vi "SweepCtrlConstCurrent_ver1.0.vi"(7 "Keithley 6221":T1={"Delta "=FALSE, "Const I "=FALSE, "Pulse Delta "=FALSE, "Sine Wave "=FALSE, "From I_HI (A)"=0.0, "From I (A)"=0.0, "I_LO (A)"=0.0, "From I_H (A)"=0.0, "I_L (A)"=0.0, "Freq (Hz)"=13.259, "From I_Sin (A)"=0.0, "DC Offset (A)"=0.0, "Delay Time (s)"=1.0, "Pulse Width (s)"=0.012, "Delay (s)"=0.011966, "To I (A)"=0.0, "ASymmetric?"=FALSE, "To I_HI (A)"=0.0, "To I_H (A)"=0.0, "To I_Sin (A)"=0.0, "GPIB ADR"=0, "Sweep Mode"=0, "Delta Unit"="V", "2182A range (V)"=0.01, "6221 Compliance (V)"=10.0} {"Sweep Mode" items=["Linear", "Log", "Exp", "Inverse", "Manual"]; "GPIB ADR" items=["None"=0, "12"=12, "13"=13]; "To I_Sin (A)" format="%#.5p"; "To I_H (A)" format="%#.5p"; "To I_HI (A)" format="%#.5p"; "To I (A)" format="%#.5p"; "Delay (s)" format="%.3p"; "Pulse Width (s)" format="%.3p"; "Delay Time (s)" format="%#.5p"; "DC Offset (A)" format="%#.5p"; "From I_Sin (A)" format="%#.5p"; "Freq (Hz)" format="%#_6p"; "I_L (A)" format="%#.5p"; "From I_H (A)" format="%#.5p"; "I_LO (A)" format="%#.5p"; "From I (A)" format="%#.5p"; "From I_HI (A)" format="%#.5p"}, 8 "error in (no error)":errorcluster, 9 "Set pt change flag":bool, 10 "DC St. Pt.":dbl, 11 "GPIB ADR":u16) -> (0 "error out":errorcluster)   [LabVIEW 2012]
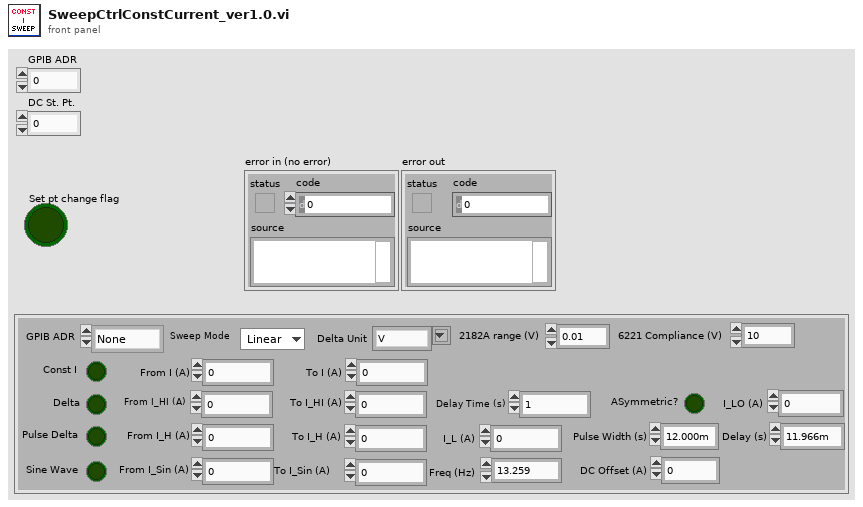
[diagram p1: front panel]
types:
  T1 = cluster{"Delta ":bool, "Const I ":bool, "Pulse Delta ":bool, "Sine Wave ":bool, "From I_HI (A)":dbl, "From I (A)":dbl, "I_LO (A)":dbl, "From I_H (A)":dbl, "I_L (A)":dbl, "Freq (Hz)":dbl, "From I_Sin (A)":dbl, "DC Offset (A)":dbl, "Delay Time (s)":dbl, "Pulse Width (s)":dbl, "Delay (s)":dbl, "To I (A)":dbl, "ASymmetric?":bool, "To I_HI (A)":dbl, "To I_H (A)":dbl, "To I_Sin (A)":dbl, "GPIB ADR":u16, "Sweep Mode":u8, "Delta Unit":string, "2182A range (V)":dbl, "6221 Compliance (V)":dbl}
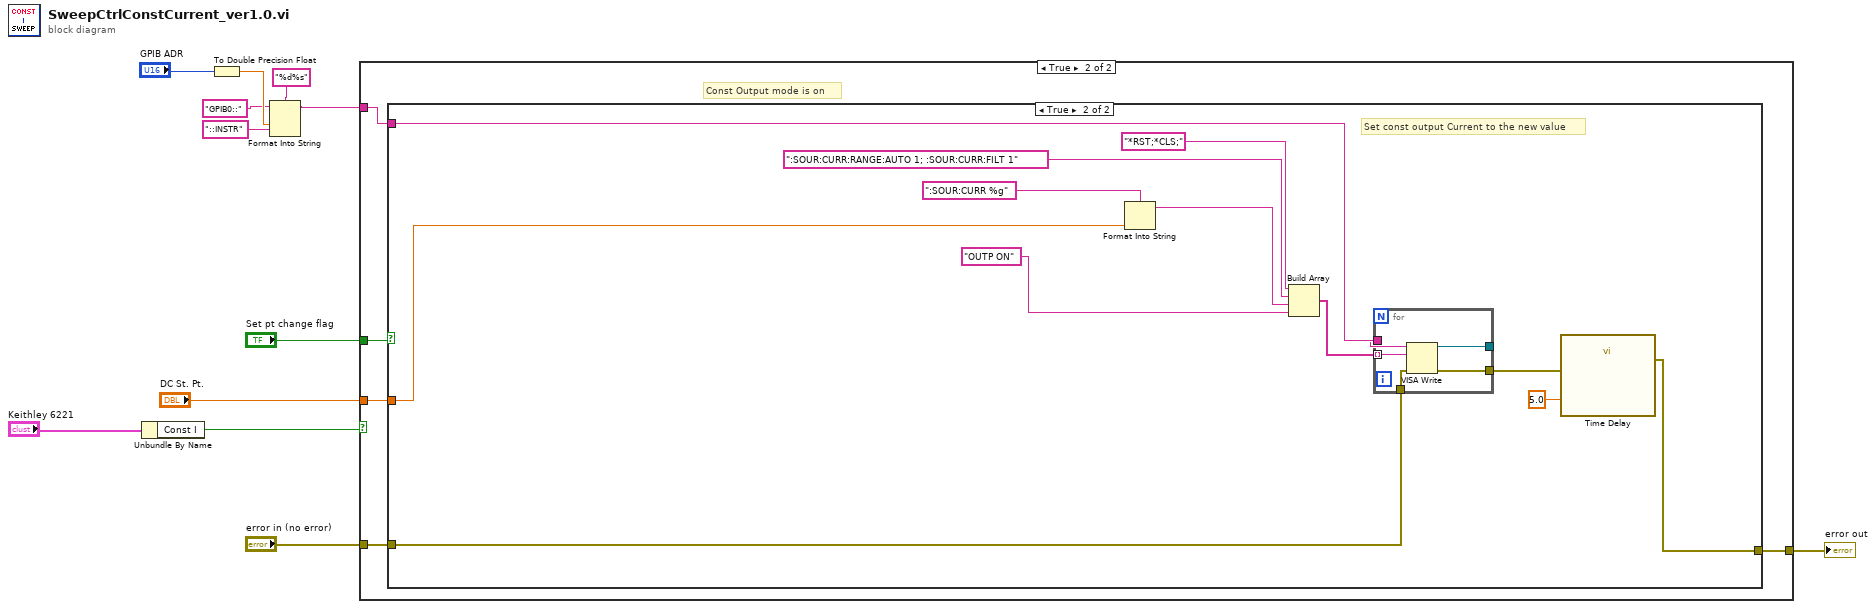
[diagram p0: block diagram]
diagram:
  n1 = Unbundle By Name("Keithley 6221") -> ("Const I"=w7:bool)
  n2 = To Double Precision Float(number="GPIB ADR") -> (double precision float=w11:dbl)
  n3 = Format Into String(format string="%d%s" ("Removes all labels from the string"), initial string="GPIB0::", w11, "::INSTR") -> (resulting string=w6:string)  [unwired: 1 in, 1 out]
  n4 = case shown="True" w7 {
    tunnel: "Set pt change flag" -> [_ w18]
    tunnel: w6 -> [_ w17]
    tunnel: "DC St. Pt." -> [_ w16]
    tunnel: "error in (no error)" -> [w13 w15]
    tunnel: [w13 w14] -> w3
    frame False {
      # "Delta mode is off"
    }
    frame True {
      # "Const Output mode is on"
      n5 = case shown="True" w18 {
        tunnel: w17 -> [_ w31]
        tunnel: w16 -> [_ w21]
        tunnel: w15 -> [w19 w28]
        tunnel: [w19 w24] -> w14
        frame False {
          # "Set Values are not changed"
        }
        frame True {
          # "Set const output Current to the new value"
          n6 = Format Into String(format string=":SOUR:CURR %g", w21) -> (resulting string=w27:string)  [unwired: 2 in, 1 out]
          n7 = Build Array("*RST;*CLS;" ("write buffer"), ":SOUR:CURR:RANGE:AUTO 1; :SOUR:CURR:FILT 1" ("write buffer"), w27, "OUTP ON" ("format string")) -> (w29:string[])
          n8 = for {
            tunnel: w29 -> [w36] mode=indexing
            tunnel: w31 -> [w35]
            tunnel: [w34] -> w25
            tunnel: w28 -> [w33]
            tunnel: [w32] -> _
            n9 = VISA Write(VISA resource name=w35, write buffer=w36, error in (no error)=w33) -> (VISA resource name out=w32:refnum<visa-resource-name>, error out=w34:errorcluster)  [unwired: 1 out]
          }
          n10 = call "Time Delay"("error in (no error)"=w25, "Delay Time (s)"=5.0) -> ("error out"=w24:errorcluster)  [unwired: 9 in]
        }
      }
    }
  }
  "error out" <- w3
